vi "LL Ring.vi"() -> ()   [LabVIEW 2013]
doc: "The LL Ring VI acquires images continuously and displays them in an image control using the low-level acquisition VIs. A ring initiates a continuous high-speed acquisition to multiple buffers and is appropriate for high-speed applications that perform processing on every image. Multiple buffers are useful when processing times vary depending on other applications and processing results .\n\nIMAQ Init initializes the device. IMAQ Configure List configures the buffer list with multiple buffers. IMAQ Create creates the image buffers. Call IMAQ Configure Buffer once for each buffer in the buffer list. IMAQ Start starts the acquisition, and IMAQ Extract Buffer ensures that the current image is not overwritten. An image control displays the image on the front panel. After exiting the loop, IMAQ Extract Buffer releases the last extracted buffer. IMAQ Close releases resources associated with the acquisition, and IMAQ Dispose frees the image buffer."
uses:
  <vilib>/vision/Image Controls.llb/IMAQ Image.ctl
panel:
  out "size(s)":i32
  in  "total images":i32=100000
  out "Frame Rate":dbl(knob) scale=0.0..10000.0
  in  "Stop":bool
  out "Last Valid Buffer":i32
  out "Image":T1(plugin-control)
  in  "Interface Name":string="img0"
  in  "Number of Images":u32=10
  # "Overview: Demonstrates how to acquire images continuously using a ring, and displays them in an image control using the low-level acquisition VIs. \nRequirements: Vision Acquisition Software, IMAQ frame grabber.\nInstructions: \n1. Select the IMAQ frame grabber Interface Name.\n2. Run the VI."
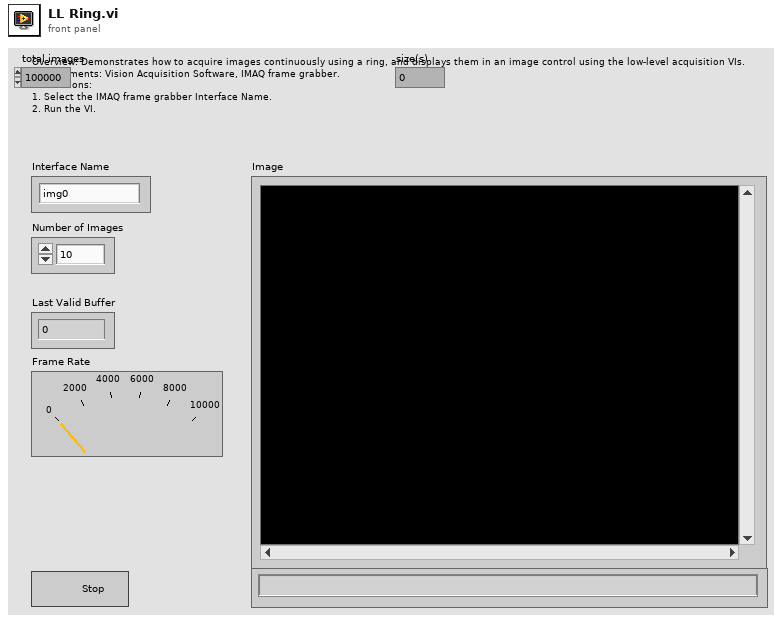
[diagram p1: front panel]
types:
  T1 = typedef "IMAQ Image.ctl" = refnum<image>
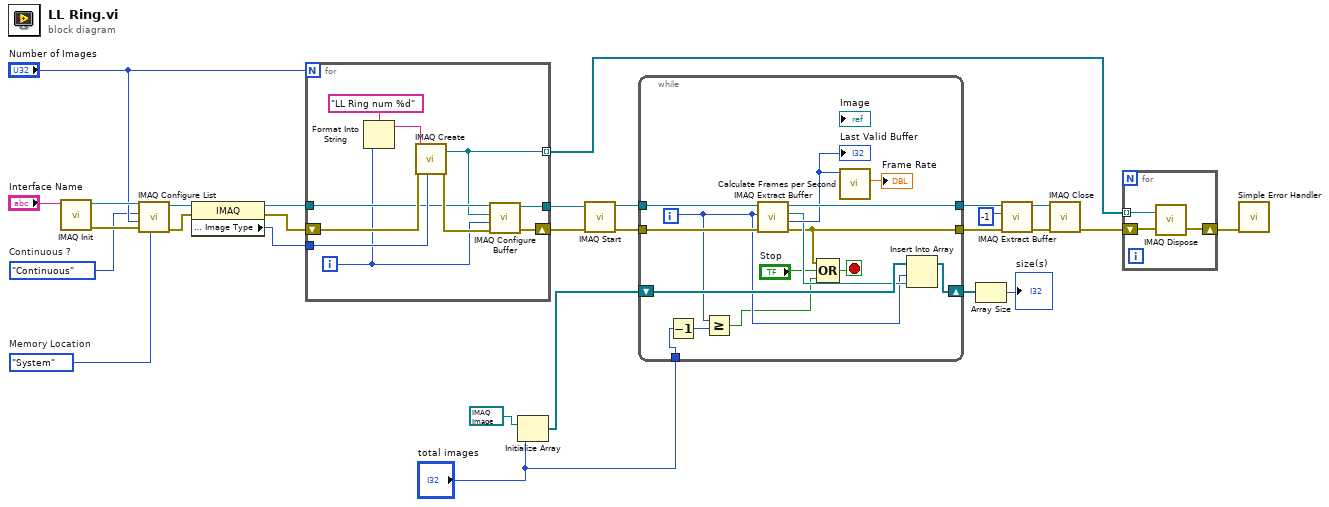
[diagram p0: block diagram]
diagram:
  w8 = enum16{"System", "Onboard"}."System"  # Memory Location
  w7 = enum16{"One-Shot", "Continuous"}."Continuous"  # Continuous ?
  n1 = call <vilib>:"IMAQ Init.vi"("Interface Name"="Interface Name") -> ("error out"=w27:errorcluster, "IMAQ Session Out"=w28:refnum<k11>)  [unwired: 1 in, 8 out]
  n2 = call <vilib>:"IMAQ Configure List.vi"("Memory Location"=w8, "error in (no error)"=w27, "Number of buffers"="Number of Images", "Continuous?"=w7, "IMAQ Session In"=w28) -> ("error out"=w23:errorcluster, "IMAQ Session Out"=w22:refnum<k11>)  [unwired: 1 in, 4 out]
  n3 = property class="IMAQ"(reference=w22, error in=w23) -> (reference out=w14:refnum<k11>, error out=w12:errorcluster, "Image Parameters : Image Type"=w13:u32)
  n4 = for {
    N: "Number of Images" -> [_]
    tunnel: [w38] -> w10
    tunnel: w13 -> [w36]
    tunnel: w14 -> [w33]
    shift-right: [w37] -> w9
    shift-left: w12 -> [w35]
    tunnel: [w29] -> w6 mode=indexing
    i -> [w30]
    n5 = Format Into String(format string="LL Ring num %d", w30) -> (resulting string=w32:string)  [unwired: 2 in, 1 out]
    n6 = call "IMAQ Create"("Image Name"=w32, "Image Type"=w36, "error in (no error)"=w35) -> ("New Image"=w29:T1, "error out"=w34:errorcluster)  [unwired: 1 in, 1 out]
    n7 = call <vilib>:"IMAQ Configure Buffer.vi"("error in (no error)"=w34, "Buffer Number"=w30, "Image In"=w29, "IMAQ Session In"=w33) -> ("error out"=w37:errorcluster, "IMAQ Session Out"=w38:refnum<k11>)  [unwired: 2 in, 4 out]
  }
  n8 = Initialize Array(T1 refnum ("Image Out"), "total images") -> (w4:T1[])
  n9 = call <vilib>:"IMAQ Start.vi"("error in (no error)"=w9, "IMAQ Session In"=w10) -> ("error out"=w18:errorcluster, "IMAQ Session Out"=w17:refnum<k11>)  [unwired: 8 out]
  n10 = while {
    tunnel: [w51] -> w20
    tunnel: w17 -> [w52]
    tunnel: w18 -> [w53]
    tunnel: [w42] -> w19
    shift-right: [w48] -> w3
    shift-left: w4 -> [w47]
    tunnel: "total images" -> [w39]
    i -> [w45]
    stop <- w44 stop-if-true
    n11 = Decrement(x=w39) -> (x-1=w40:i32)
    n12 = Greater Or Equal?(x=w45, y=w40) -> (x >= y?=w41:bool)
    n13 = call <vilib>:"IMAQ Extract Buffer.vi"("error in (no error)"=w53, "Buffer to extract"=w45, "IMAQ Session In"=w52) -> ("error out"=w42:errorcluster, "Buffer Number"=w49:i32, "Image Out"=w46:T1, "IMAQ Session Out"=w51:refnum<k11>)  [unwired: 5 out]
    "Last Valid Buffer" <- w49
    n14 = Compound Arithmetic op=OR(w42, "Stop", w41) -> (w44:bool)
    n15 = call <vilib>:"Calculate Frames per Second.vi"("Buffer Number"=w49) -> ("Processed Frames/s"=→"Frame Rate":dbl)  [unwired: 8 in, 2 out]
    n16 = Insert Into Array(array=w47, index=w45, new element=w46) -> (w48:T1[])
  }
  n17 = Array Size(array=w3) -> (size(s)=→"size(s)":i32)
  n18 = call <vilib>:"IMAQ Extract Buffer.vi"("error in (no error)"=w19, "Buffer to extract"=-1, "IMAQ Session In"=w20) -> ("error out"=w16:errorcluster, "IMAQ Session Out"=w15:refnum<k11>)  [unwired: 7 out]
  n19 = call <vilib>:"IMAQ Close.vi"("error in (no error)"=w16, "IMAQ Session In"=w15) -> ("error out"=w24:errorcluster)  [unwired: 9 out]
  n20 = for {
    tunnel: w6 -> [w56] mode=indexing
    shift-right: [w54] -> w25
    shift-left: w24 -> [w55]
    n21 = call "IMAQ Dispose"("Image"=w56, "error in (no error)"=w55) -> ("error out"=w54:errorcluster)  [unwired: 1 in, 3 out]
  }
  n22 = call <vilib>:"Simple Error Handler.vi"("error in (no error)"=w25) -> ()  [unwired: 1 in, 8 out]
